vi "Helmholtz2D_FEM_Gen Grid.vi"(9 "grid factor":dbl, 10 "Y":dbl[](array[numeric]), 11 "X":dbl[](array[numeric])) -> (2 "Yi":dbl[](array[numeric]), 3 "Xi":dbl[](array[numeric]))   [LabVIEW 2020, in "NI_PDE.lvlib"]
uses:
  <vilib>/gmath/NI_PDE.lvlib
  <vilib>/Analysis/1siggen.llb/Ramp Pattern by Samples.vi
  <vilib>/Analysis/NI_AALBase.lvlib
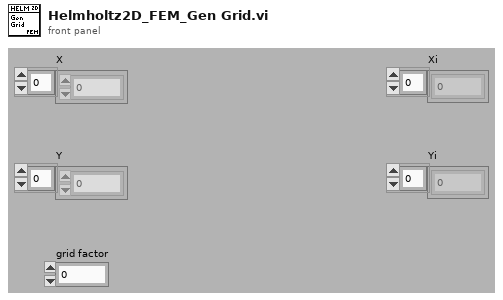
[diagram p1: front panel]
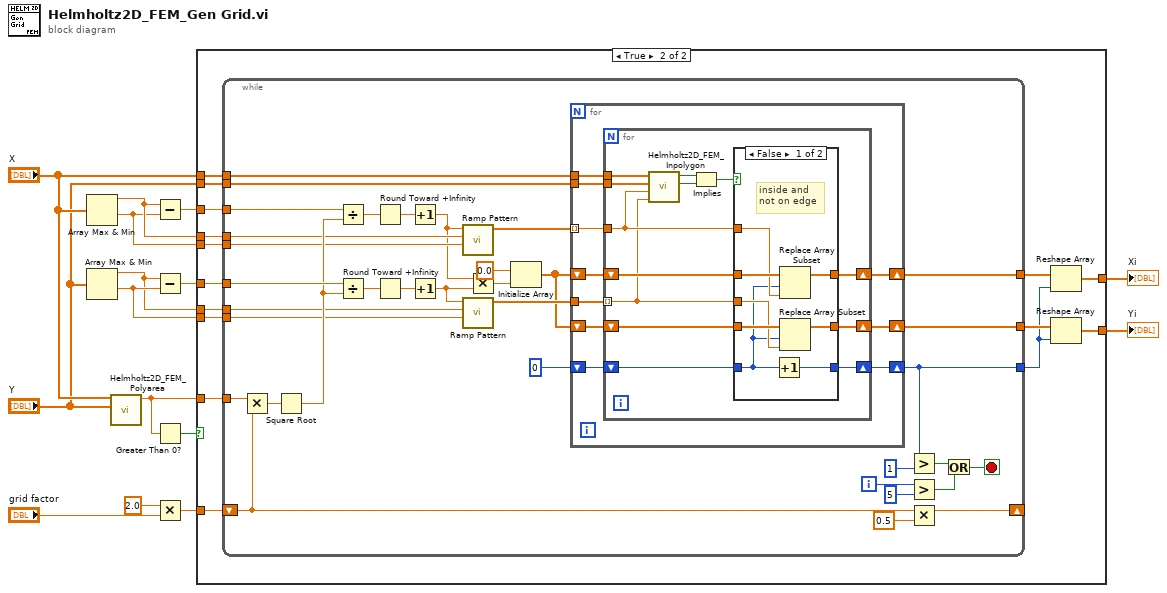
[diagram p0: block diagram]
diagram:
  n1 = Array Max & Min(array="X") -> (max value=w10:dbl, min value=w9:dbl)  [unwired: 2 out]
  n2 = Array Max & Min(array="Y") -> (max value=w7:dbl, min value=w8:dbl)  [unwired: 2 out]
  n3 = call <vilib>:"Helmholtz2D_FEM_Polyarea.vi"("Y"="Y", "X"="X") -> ("area"=w4:dbl)  [unwired: 9 out]
  n4 = Subtract(x=w10, y=w9) -> (x-y=w12:dbl)
  n5 = Subtract(x=w7, y=w8) -> (x-y=w11:dbl)
  n6 = Greater Than 0?(x=w4) -> (x > 0?=w3:bool)
  n7 = Multiply(x=2.0, y="grid factor") -> (x*y=w13:dbl)
  n8 = case shown="True" w3 {
    tunnel: w13 -> [_ w30]
    tunnel: w12 -> [_ w29]
    tunnel: w11 -> [_ w28]
    tunnel: w10 -> [_ w27]
    tunnel: w9 -> [_ w26]
    tunnel: w8 -> [_ w25]
    tunnel: w7 -> [_ w24]
    tunnel: "X" -> [_ w23]
    tunnel: "Y" -> [_ w22]
    tunnel: [_ w20] -> w6
    tunnel: [_ w17] -> w5
    tunnel: w4 -> [_ w16]
    frame False {
    }
    frame True {
      n9 = while {
        tunnel: w16 -> [w65]
        tunnel: w29 -> [w63]
        tunnel: w28 -> [w62]
        tunnel: w27 -> [w56]
        tunnel: w26 -> [w55]
        tunnel: w25 -> [w54]
        tunnel: w24 -> [w53]
        tunnel: w23 -> [w52]
        tunnel: w22 -> [w51]
        tunnel: [w42] -> w21
        tunnel: [w41] -> w19
        tunnel: [w40] -> w18
        shift-right: [w36] -> _
        shift-left: w30 -> [w37]
        i -> [w34]
        stop <- w33 stop-if-true
        n10 = Multiply(x=w65, y=w37) -> (x*y=w64:dbl)
        n11 = Square Root(x=w64) -> (sqrt(x)=w61:dbl)
        n12 = Divide(x=w63, y=w61) -> (x/y=w60:dbl)
        n13 = Divide(x=w62, y=w61) -> (x/y=w57:dbl)
        n14 = Round Toward +Infinity(x=w60) -> (ceil(x): smallest int >= x=w59:dbl)
        n15 = Round Toward +Infinity(x=w57) -> (ceil(x): smallest int >= x=w58:dbl)
        n16 = Increment(x=w59) -> (x+1=w48:dbl)
        n17 = Increment(x=w58) -> (x+1=w47:dbl)
        n18 = call-poly <vilib>:"Ramp Pattern.vi"("start"=w55, "end"=w56, "samples"=w48) -> ("Ramp Pattern"=w50:dbl[])  [unwired: 7 in, 1 out]
        n19 = call-poly <vilib>:"Ramp Pattern.vi"("start"=w54, "end"=w53, "samples"=w47) -> ("Ramp Pattern"=w49:dbl[])  [unwired: 7 in, 1 out]
        n20 = Multiply(x=w48, y=w47) -> (x*y=w46:dbl)
        n21 = Initialize Array(0.0 ("element"), w46) -> (w44:dbl[])
        n22 = for {
          tunnel: w52 -> [w75]
          tunnel: w51 -> [w74]
          tunnel: w50 -> [w73] mode=indexing
          tunnel: w49 -> [w72]
          shift-right: [w69] -> w42
          shift-left: w44 -> [w70]
          shift-right: [w68] -> w41
          shift-left: w44 -> [w71]
          shift-right: [w66] -> w40
          shift-left: 0 -> [w67]
          n23 = for {
            tunnel: w75 -> [w88]
            tunnel: w74 -> [w87]
            tunnel: w73 -> [w86]
            tunnel: w72 -> [w84] mode=indexing
            shift-right: [w81] -> w68
            shift-left: w71 -> [w83]
            shift-right: [w82] -> w69
            shift-left: w70 -> [w85]
            shift-right: [w79] -> w66
            shift-left: w67 -> [w80]
            n24 = call <vilib>:"Helmholtz2D_FEM_Inpolygon.vi"("yi"=w84, "xi"=w86, "Y"=w87, "X"=w88) -> ("on edge?"=w78:bool, "inside?"=w77:bool)  [unwired: 6 out]
            n25 = Implies(1:w78, 2:w77) -> (0:w76:bool)
            n26 = case shown="False" w76 {
              tunnel: w86 -> [w95 _]
              tunnel: w85 -> [w96 w99]
              tunnel: w84 -> [w93 _]
              tunnel: w83 -> [w94 w98]
              tunnel: [w92 w99] -> w82
              tunnel: [w91 w98] -> w81
              tunnel: w80 -> [w90 w97]
              tunnel: [w89 w97] -> w79
              frame False {
                # "inside and\nnot on edge"
                n27 = Increment(x=w90) -> (x+1=w89:i32)
                n28 = Replace Array Subset(array=w96, new element=w95, index=w90) -> (w92:dbl[])
                n29 = Replace Array Subset(array=w94, new element=w93, index=w90) -> (w91:dbl[])
              }
              frame True {
              }
            }
          }
        }
        n30 = Greater?(x=w40, y=1) -> (0:w39:bool)
        n31 = Greater?(x=w34, y=5) -> (0:w32:bool)
        n32 = Multiply(x=w37, y=0.5) -> (x*y=w36:dbl)
        n33 = Or(x=w39, y=w32) -> (x .or. y?=w33:bool)
      }
      n34 = Reshape Array(w21, w18) -> (w20:dbl[])
      n35 = Reshape Array(w19, w18) -> (w17:dbl[])
    }
  }
  "Xi" <- w6
  "Yi" <- w5
